vi "limits with distance.vi"(8 "distanceM3":dbl, 9 "distanceM2":dbl, 10 "distanceM1":dbl, 11 "cluster":T1) -> (0 "M3 Distance":dbl, 1 "M2 Distance":dbl, 2 "M1 Distance":dbl)   [LabVIEW 2012]
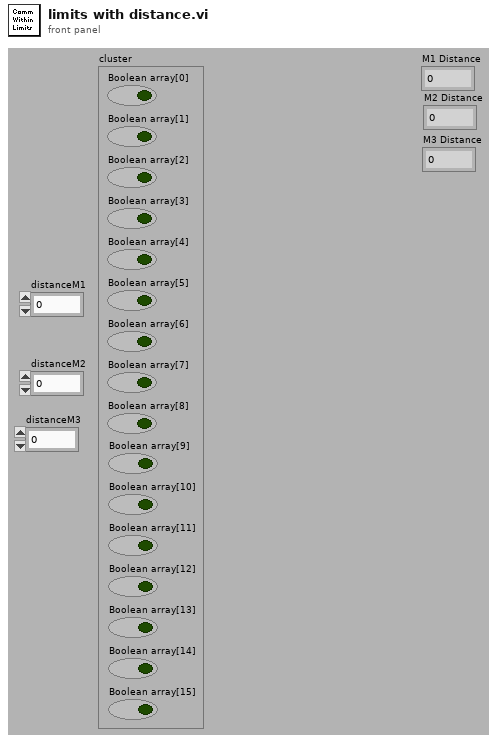
[diagram p1: front panel]
types:
  T1 = cluster{"Boolean array[0]":bool, "Boolean array[1]":bool, "Boolean array[2]":bool, "Boolean array[3]":bool, "Boolean array[4]":bool, "Boolean array[5]":bool, "Boolean array[6]":bool, "Boolean array[7]":bool, "Boolean array[8]":bool, "Boolean array[15]":bool, "Boolean array[14]":bool, "Boolean array[13]":bool, "Boolean array[12]":bool, "Boolean array[11]":bool, "Boolean array[10]":bool, "Boolean array[9]":bool}
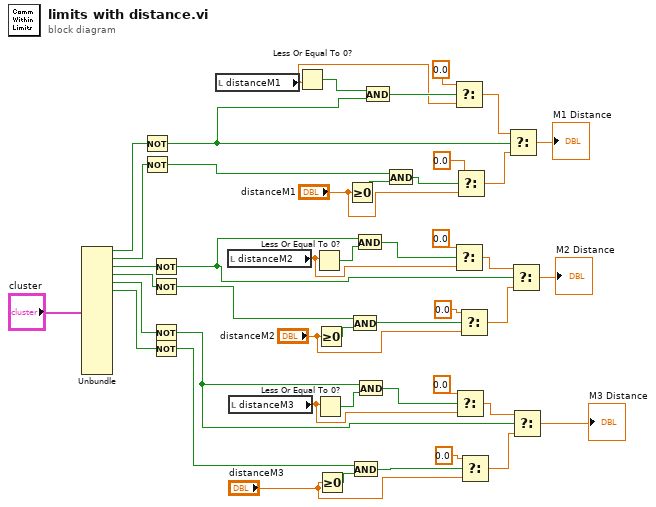
[diagram p0: block diagram]
diagram:
  n1 = Unbundle("cluster") -> ("Boolean array[0]"=w45:bool, "Boolean array[1]"=w43:bool, "Boolean array[2]"=w44:bool, "Boolean array[3]"=w46:bool, "Boolean array[4]"=w7:bool, "Boolean array[5]"=w6:bool)  [unwired: 10 out]
  n2 = Not(x=w45) -> (.not. x?=w5:bool)
  n3 = Not(x=w43) -> (.not. x?=w20:bool)
  n4 = Not(x=w44) -> (.not. x?=w2:bool)
  n5 = Not(x=w46) -> (.not. x?=w4:bool)
  n6 = Not(x=w7) -> (.not. x?=w1:bool)
  n7 = Not(x=w6) -> (.not. x?=w3:bool)
  n8 = local read "distanceM1"() -> (w40:dbl)
  n9 = local read "distanceM2"() -> (w30:dbl)
  n10 = local read "distanceM3"() -> (w15:dbl)
  n11 = Less Or Equal To 0?(x=w40) -> (x <= 0?=w42:bool)
  n12 = Less Or Equal To 0?(x=w30) -> (x <= 0?=w33:bool)
  n13 = Less Or Equal To 0?(x=w15) -> (x <= 0?=w18:bool)
  n14 = Greater Or Equal To 0?(x="distanceM2") -> (x >= 0?=w28:bool)
  n15 = Greater Or Equal To 0?(x="distanceM3") -> (x >= 0?=w13:bool)
  n16 = Greater Or Equal To 0?(x="distanceM1") -> (x >= 0?=w19:bool)
  n17 = And(x=w4, y=w28) -> (x .and. y?=w27:bool)
  n18 = And(x=w3, y=w13) -> (x .and. y?=w12:bool)
  n19 = And(x=w2, y=w33) -> (x .and. y?=w32:bool)
  n20 = And(x=w1, y=w18) -> (x .and. y?=w17:bool)
  n21 = And(x=w42, y=w5) -> (x .and. y?=w41:bool)
  n22 = And(x=w20, y=w19) -> (x .and. y?=w37:bool)
  n23 = Select(t=0.0, s=w41, f=w40) -> (s? t:f=w38:dbl)
  n24 = Select(t=0.0, s=w32, f=w30) -> (s? t:f=w29:dbl)
  n25 = Select(t=0.0, s=w17, f=w15) -> (s? t:f=w14:dbl)
  n26 = Select(t=0.0, s=w37, f="distanceM1") -> (s? t:f=w34:dbl)
  n27 = Select(t=0.0, s=w27, f="distanceM2") -> (s? t:f=w24:dbl)
  n28 = Select(t=0.0, s=w12, f="distanceM3") -> (s? t:f=w10:dbl)
  n29 = Select(t=w38, s=w5, f=w34) -> (s? t:f=→"M1 Distance":dbl)
  n30 = Select(t=w29, s=w2, f=w24) -> (s? t:f=→"M2 Distance":dbl)
  n31 = Select(t=w14, s=w1, f=w10) -> (s? t:f=→"M3 Distance":dbl)
